vi "Event UI.vi"(8 "error in (no error)":errorcluster, 11 "Wait Event in":refnum<class "Wait Event.lvclass">) -> (0 "error out":errorcluster, 3 "Wait Event out":refnum<class "Wait Event.lvclass">)   [LabVIEW 2018, in "Wait Event.lvclass"]
uses:
  Wait Event.lvclass
  State/State.lvclass
  User State 1/User State 1.lvclass
  C:/Users/fflores/Documents/OOP-State-Machine/State/State.lvclass
  User State 2/User State 2.lvclass
  Exit/Exit.lvclass
panel:
  in  "Do Something Else <Replace Me>":bool
  in  "Do Something <Replace Me>":bool
  in  "Exit":bool
  # "These controls have associated \"Value Changed\" events configured in the Event Structure on the diagram.\n\nReplace them (and reconfigure the Event Structure) with the controls you need for your application."
  # "This template is for the Simple State Machine design pattern.\n\nSee the block diagram for more information on how to use this template."
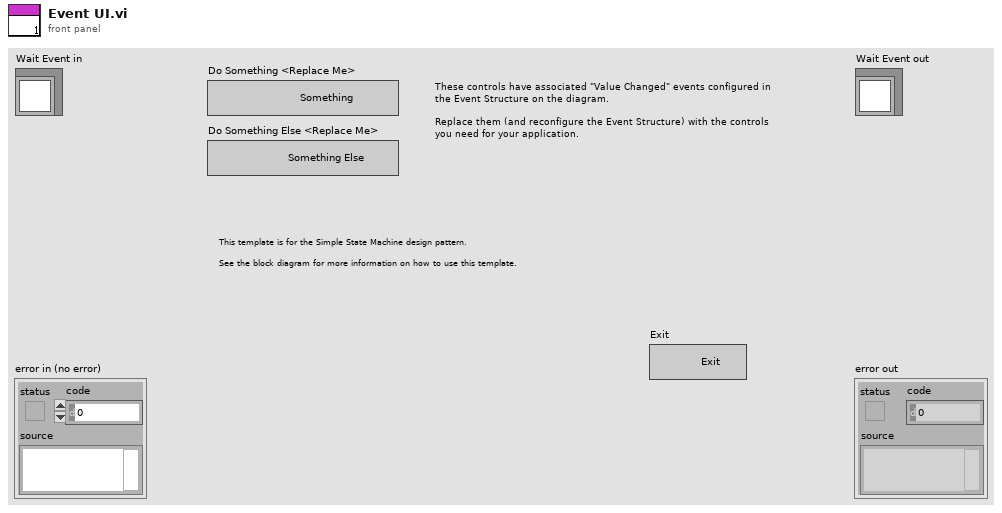
[diagram p1: front panel]
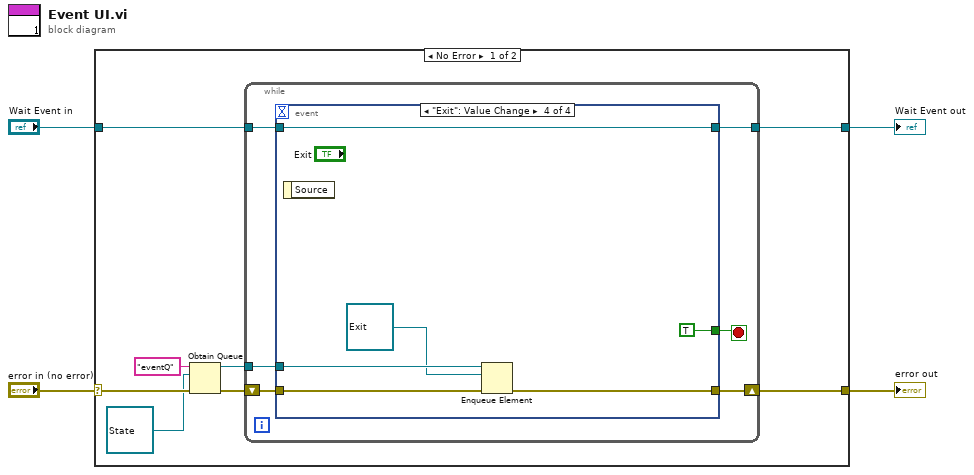
[diagram p0: block diagram]
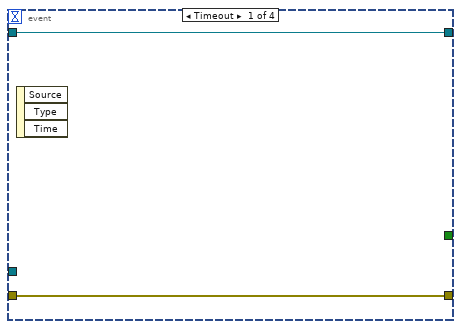
[diagram p2: hidden frame]
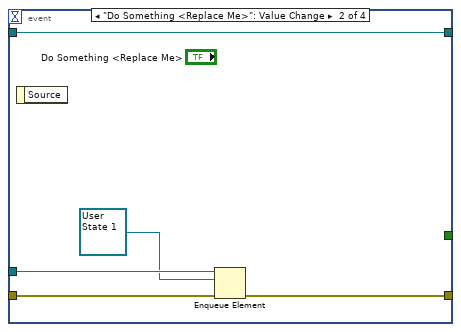
[diagram p3: hidden frame]
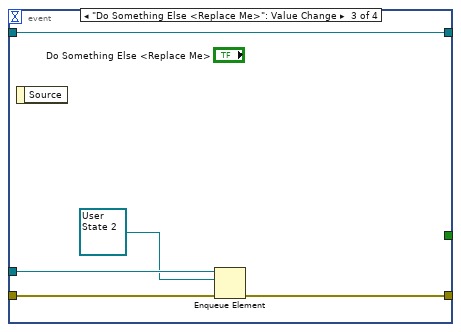
[diagram p4: hidden frame]
diagram:
  n1 = case shown="No Error" "error in (no error)" {
    selector: "error in (no error)" -> [w10 w38]
    tunnel: [w9 w38] -> w3
    tunnel: [w11 w37] -> w1
    tunnel: "Wait Event in" -> [w12 w37]
    frame No Error {
      n2 = Obtain Queue(name (unnamed)="eventQ", element data type=refnum<class "State.lvclass"> refnum ("State.lvclass"), error in (no error)=w10) -> (queue out=w5:refnum<queue>, error out=w8:errorcluster)  [unwired: 2 in, 1 out]
      n3 = while {
        tunnel: w12 -> [w18]
        tunnel: [w17] -> w11
        shift-right: [w15] -> w9
        shift-left: w8 -> [w16]
        tunnel: w5 -> [w14]
        stop <- w13 stop-if-true
        n4 = event shown="[3] \"Exit\": Value Change" {
          selector: _ -> [_ _ _ _]
          dyn-events: _ -> [_ _ _ _]
          timeout: _ -> [_ _ _ _]
          tunnel: w18 -> [w20 w25 w30 w36]
          tunnel: [w20 w25 w30 w36] -> w17
          tunnel: w16 -> [w19 w24 w29 w35]
          tunnel: [w19 w23 w28 w34] -> w15
          tunnel: w14 -> [_ w22 w27 w33]
          tunnel: [_ _ _ TRUE] -> w13
          event Timeout {
            n5 = event-data() -> ()  [unwired: 1 in, 3 out]
          }
          event "Do Something <Replace Me>": Value Change {
            n6 = event-data() -> ()  [unwired: 1 in, 1 out]
            n7 = Enqueue Element(queue=w22, element=refnum<class "User State 1.lvclass"> refnum ("User State 1.lvclass"), error in (no error)=w24) -> (error out=w23:errorcluster)  [unwired: 1 in, 2 out]
          }
          event "Do Something Else <Replace Me>": Value Change {
            n8 = event-data() -> ()  [unwired: 1 in, 1 out]
            n9 = Enqueue Element(queue=w27, element=refnum<class "User State 2.lvclass"> refnum ("User State 2.lvclass"), error in (no error)=w29) -> (error out=w28:errorcluster)  [unwired: 1 in, 2 out]
          }
          event "Exit": Value Change {
            n10 = event-data() -> ()  [unwired: 1 in, 1 out]
            n11 = Enqueue Element(queue=w33, element=refnum<class "Exit.lvclass"> refnum ("Stop.lvclass"), error in (no error)=w35) -> (error out=w34:errorcluster)  [unwired: 1 in, 2 out]
          }
        }
      }
    }
    frame Error {
    }
  }
  "error out" <- w3
  "Wait Event out" <- w1
